vi "Import Configuration.vi"(8 "error in (no error)":errorcluster, 11 "Node Ptr":u64 format="%.0x") -> (0 "error out":errorcluster)   [LabVIEW 2014, in "SLSC configuration System Explorer.lvlib"]
uses:
  SLSC configuration System Explorer.lvlib
  C:/Files/Custom VeriStand Development/DET-SPI-Tool/XML Deserializer/SLSC Deserializer/SLSC Deserializer/bin/Release/SLSC Deserializer.dll
  XML Deserializer/SLSC Deserializer/SLSC Deserializer/bin/Release/SLSC Deserializer.dll
  <vilib>/NI Veristand/Custom Device API/Custom Device API.lvlib
  <vilib>/NI Veristand/Custom Device Tools/Custom Device Utility Library/Custom Device Utility Library.lvlib
panel:
  in  "Cancel":bool
  in  "OK":bool
  in  "XML Import Path":path
  in  "Tag":string
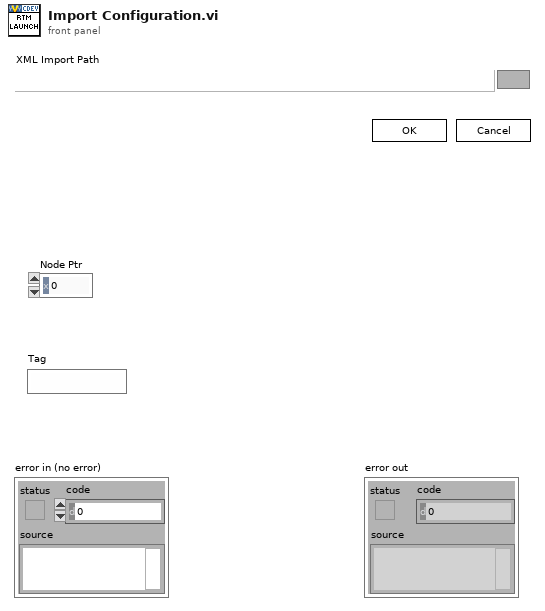
[diagram p1: front panel]
types:
  T1 = enum8{"Enabled", "Disabled", "Disabled and Grayed Out"}
  T2 = typedef "Custom Device API.lvlib/Custom Device Item Ref.ctl" = u64
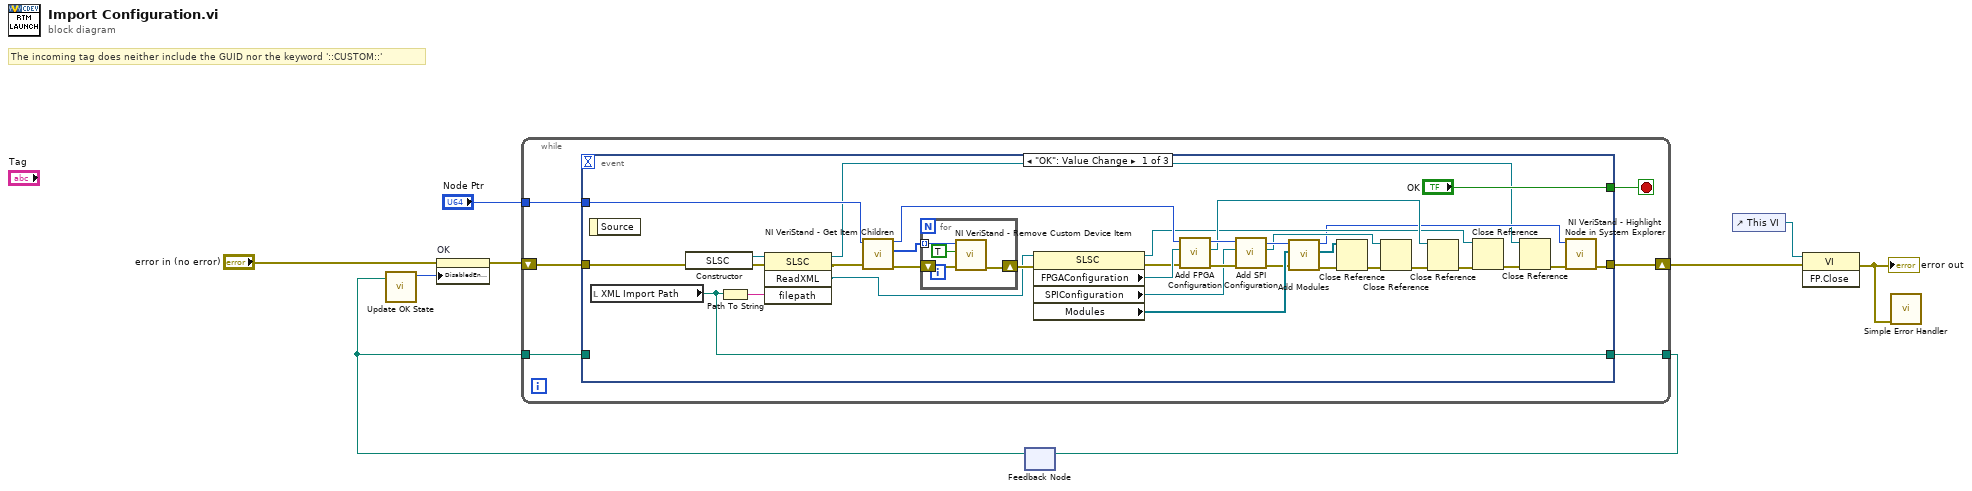
[diagram p0: block diagram]
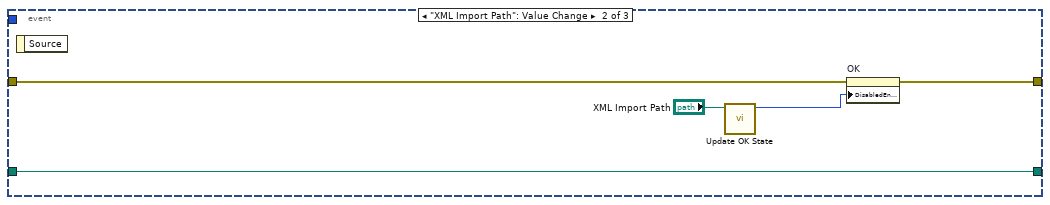
[diagram p2: hidden frame]
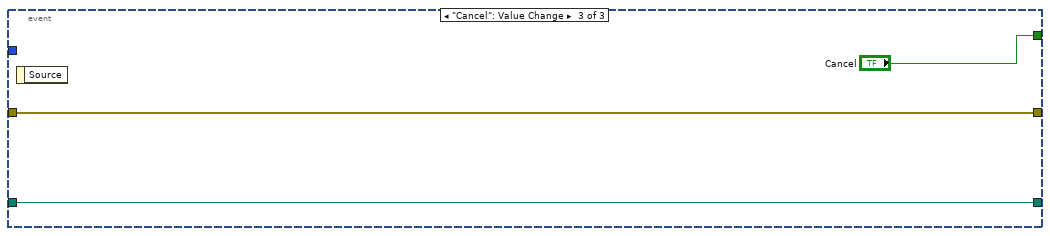
[diagram p3: hidden frame]
diagram:
  # "The incoming tag does neither include the GUID nor the keyword '::CUSTOM::'"
  n1 = feedback #1() -> (w2:path)  [unwired: 1 in]
  n2 = call "Update OK State.vi"("XML Export Path"=w2) -> ("OK State"=w9:T1)  [unwired: 10 in]
  n3 = property on="OK" class="Bool"(error in="error in (no error)", "DisabledEnum"=w9) -> (error out=w6:errorcluster)  [unwired: 1 in, 1 out]
  n4 = while {
    shift-right: [w13] -> w4
    shift-left: w6 -> [w15]
    tunnel: "Node Ptr" -> [w12]
    tunnel: [w11] -> w3
    tunnel: w2 -> [w10]
    stop <- w14 stop-if-true
    n5 = event shown="[0] \"OK\": Value Change" {
      selector: _ -> [_ _ _]
      dyn-events: _ -> [_ _ _]
      timeout: _ -> [_ _ _]
      tunnel: w15 -> [w48 w55 w61]
      tunnel: ["OK" _ "Cancel"] -> w14
      tunnel: [w26 w58 w61] -> w13
      tunnel: w12 -> [w37 _ _]
      tunnel: [w25 w54 w59] -> w11
      tunnel: w10 -> [_ w54 w59]
      event "OK": Value Change {
        n6 = event-data() -> ()  [unwired: 1 in, 1 out]
        n7 = local read "XML Import Path"() -> (w25:path)
        n8 = constructor class="SLSC"(error in=w48) -> (reference out=w20:refnum<k24>, error out=w21:errorcluster)  [unwired: 2 in, 1 out]
        n9 = Path To String(path=w25) -> (string=w19:string)
        n10 = invoke class="SLSC" method="ReadXML"(reference=w20, error in=w21, "filepath"=w19) -> (reference out=w17:refnum<k24>, error out=w18:errorcluster, "ReadXML"=w16:refnum<k24>)  [unwired: 1 in, 1 out]
        n11 = call <vilib>:"NI VeriStand - Get Item Children.vi"("error in (no error)"=w18, "Item Ref in"=w37) -> ("error out"=w44:errorcluster, "Child Refs"=w43:T2[], "Item Ref out"=w30:T2)  [unwired: 6 in, 1 out]
        n12 = for {
          tunnel: w43 -> [w52] mode=indexing
          shift-right: [w53] -> w22
          shift-left: w44 -> [w51]
          n13 = call <vilib>:"NI VeriStand - Remove Custom Device Item.vi"("error in (no error)"=w51, "Force Delete (F)"=TRUE, "Item Ref in"=w52) -> ("error out"=w53:errorcluster)  [unwired: 7 in, 1 out]
        }
        n14 = property class="SLSC"(reference=w16, error in=w22) -> (reference out=w28:refnum<k24>, error out=w38:errorcluster, "FPGAConfiguration"=w39:refnum<k24>, "SPIConfiguration"=w40:refnum<k24>, "Modules"=w46:refnum<k24>[])
        n15 = call "Add FPGA Configuration.vi"("error in (no error)"=w38, "FPGA Configuration in"=w39, "Item Ref in"=w30) -> ("error out"=w41:errorcluster, "FPGA Configuration out"=w31:refnum<k24>, "Item Ref out"=w42:T2)  [unwired: 6 in]
        n16 = call "Add SPI Configuration.vi"("error in (no error)"=w41, "SPI Configuration in"=w40, "Item Ref in"=w42) -> ("error out"=w45:errorcluster, "SPI Configuration out"=w33:refnum<k24>, "Item Ref out"=w47:T2)  [unwired: 6 in]
        n17 = call "Add Modules.vi"("error in (no error)"=w45, "Modules in"=w46, "Item Ref in"=w47) -> ("error out"=w36:errorcluster, "Modules out"=w35:refnum<k24>[], "Item Ref out"=w27:T2)  [unwired: 6 in]
        n18 = Close Reference(reference=w35, error in (no error)=w36) -> (error out=w34:errorcluster)
        n19 = Close Reference(reference=w33, error in (no error)=w34) -> (error out=w32:errorcluster)
        n20 = Close Reference(reference=w31, error in (no error)=w32) -> (error out=w29:errorcluster)
        n21 = Close Reference(reference=w28, error in (no error)=w29) -> (error out=w24:errorcluster)
        n22 = Close Reference(reference=w17, error in (no error)=w24) -> (error out=w23:errorcluster)
        n23 = call <vilib>:"NI VeriStand - Highlight Node in System Explorer.vi"("error in (no error)"=w23, "Item Ref in"=w27) -> ("error out"=w26:errorcluster)  [unwired: 8 in, 1 out]
      }
      event "XML Import Path": Value Change {
        n24 = event-data() -> ()  [unwired: 1 in, 1 out]
        n25 = call "Update OK State.vi"("XML Export Path"="XML Import Path") -> ("OK State"=w56:T1)  [unwired: 10 in]
        n26 = property on="OK" class="Bool"(error in=w55, "DisabledEnum"=w56) -> (error out=w58:errorcluster)  [unwired: 1 in, 1 out]
      }
      event "Cancel": Value Change {
        n27 = event-data() -> ()  [unwired: 1 in, 1 out]
      }
    }
  }
  n28 = feedback-in #1(w3) -> ()
  n29 = control-ref of="This VI"() -> (w7:refnum<vi>)
  n30 = invoke class="VI" method="FP.Close"(reference=w7, error in=w4) -> (error out=w1:errorcluster)  [unwired: 1 in, 2 out]
  "error out" <- w1
  n31 = call <vilib>:"Simple Error Handler.vi"("error in (no error)"=w1) -> ()  [unwired: 4 in, 5 out]
